vi "Help.vi"(8 "Error In":errorcluster) -> (0 "Error Out":errorcluster)   [LabVIEW 2017]
panel:
  in  "OK Button":bool
  # "Step 1: Create a session by selecting a deployment target (username and password if applicable) and click on Create Session.\nStep 2: Select *.mdl, *.slx, *.psimsch, *.cct or NI Multisim *.xml file. In addition, choose the eHS Form Factor for the generation and a Core Index for this model. You can use this core index throughout the application to refer to a specific model.\nStep 3: Click on Add Model to add this model to the eHS Matrix Generation session.\nStep 4: Repeat step 2 & 3 if you want to generate more then one eHS matrix.\nStep 5: Click on Extract Model(s). This can take several minutes. The information extraction results will be displayed in the consoles to the right.\nStep 6 (Optional): Press the Update Settings button to change some of the matrix generation parameters before generating them.\nStep 7: Click on Generate Matrix(s). A eHS matrix will be generated for each model that was loaded into the session.\nStep 8: Once the matrices have been generated, you can transfer the matrices to the deplayment target by clicking on the Transfer Matrices button. \nStep 9: At this point, you can update the setting and generate a new set of matrices (Update Settings), you can reset the session (Reset Session), you can close the current session (Close Session), or you can stop the application (Quit). \n \nBefore running this VI please note that:\n\n1- Before starting the real-time simulation, users need to define the circuit configuration, using an appropriate circuit editor. \nThe following circuit editors are supported by OPAL-RT TECHNOLOGIES:           \n                - Matlab/Simulink SimPowwerSystems (SPS)  (*.mdl or *.slx)\n                - Matlab/Simulink PLECS blockset  (*.mdl or *.slx)\n                - PSIM  (*.psimsch or *.cct)\n                - NI Multisim (xml output *.xml)\n\n2- PSIM and NI Multisim users have to install\t32-bit version of MATLAB® Runtime version 9.0 (R2015b) availible at:\n                                 http://www.mathworks.com/products/compiler/mcr/index.html\n\n3- Please also note that you need to have valid licence of one of the mentioned circuit editors to be able to generate the eSH matrix.\nIn other words the users who want to select SimPowerSystem (SPS) model must be have valid licence of Matlab/Simulink and SPS toolbox, the users who want to select PLECS blockset model must be have valid licence of Matlab/Simulink and PLECS blockset,                       the users who want to select PSIM model must be have valid licence of PSIM, and the users who want to generate and select the NI Multism xml file must be have valid licence of NI Multisim. If you don't have valid license of the mentioned circuit editors, you can only select prebuilt xml files."
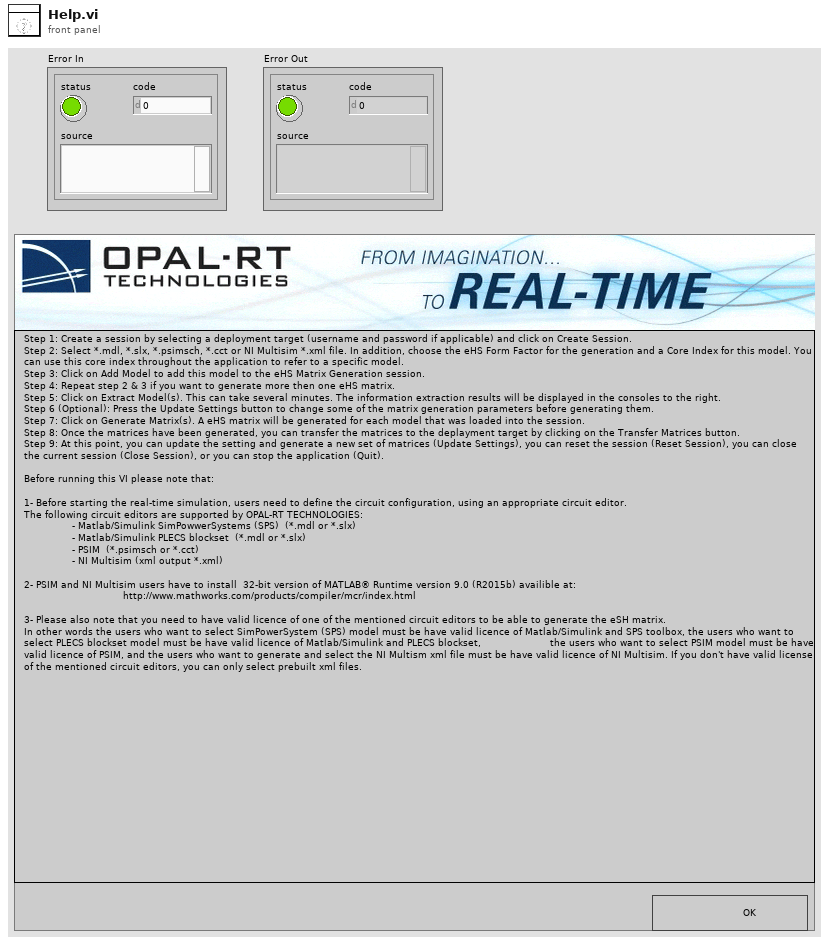
[diagram p1: front panel]
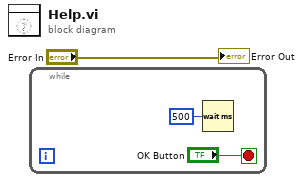
[diagram p0: block diagram]
diagram:
  n1 = while {
    stop <- "OK Button" stop-if-true
    n2 = Wait (ms)(milliseconds to wait=u32 500) -> ()  [unwired: 1 out]
  }
  "Error Out" <- "Error In"
